vi "Hold_64.vi"(8 "valid in":bool, 11 "value in":fxp<+/-,64,26>) -> (0 "valid out":bool, 3 "value out":fxp<+/-,64,26>)   [LabVIEW 2018]
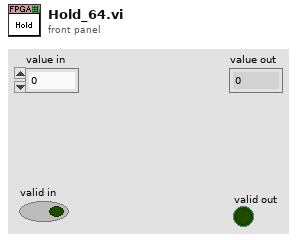
[diagram p1: front panel]
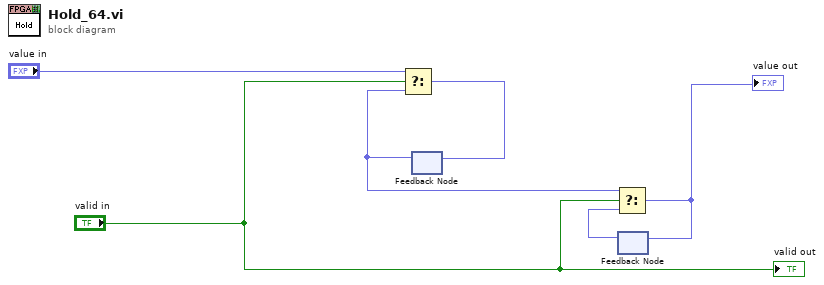
[diagram p0: block diagram]
diagram:
  n1 = feedback #1() -> (w3:fxp<+/-,64,26>)  [unwired: 1 in]
  n2 = Select(t="value in", s="valid in", f=w3) -> (s? t:f=w5:fxp<+/-,64,26>)
  n3 = feedback-in #1(w5) -> ()
  n4 = feedback #2() -> (w2:fxp<+/-,64,26>)  [unwired: 1 in]
  n5 = Select(t=w3, s="valid in", f=w2) -> (s? t:f=w1:fxp<+/-,64,26>)
  "value out" <- w1
  n6 = feedback-in #2(w1) -> ()
  "valid out" <- "valid in"
